vi "validate.vi"(8 "error in":errorcluster, 11 "Standard Engine Repo Data in":refnum<class "Standard Engine Configuration.lvclass">) -> (0 "error out":errorcluster, 3 "Standard Engine Repo Data out":refnum<class "Standard Engine Configuration.lvclass">)   [LabVIEW 2013, in "Standard Engine Configuration.lvclass"]
uses:
  Standard Engine Configuration.lvclass
  <vilib>/NI/Module Execution Interface/Engine Configuration/engine configuration.lvclass
  Standard Engine Configuration.lvclass/Standard Engine Configuration.ctl
  <vilib>/NI/CEF/CEF_TreeControl/NISE_CEF_TreeControl.lvlib
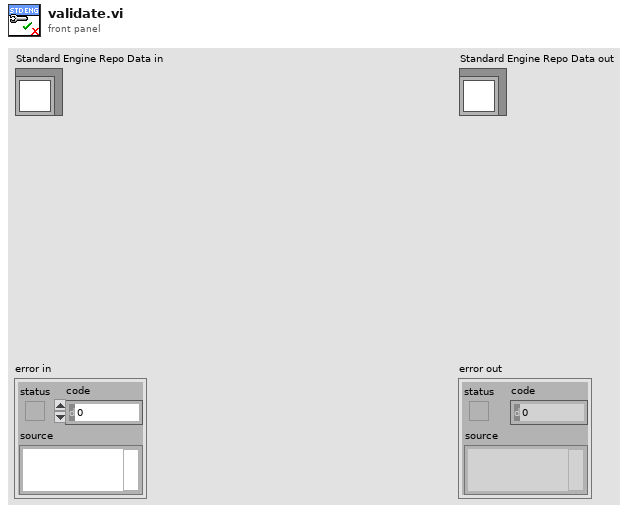
[diagram p1: front panel]
types:
  T1 = typedef "Standard Engine Configuration.lvclass/Module Specific Configuration.ctl" = cluster{"Module ID":string, "Module Decimation":T2, "Module Error Configuration":T3, "execution order priority":i32, "async?":bool, "error tag":string}
  T2 = typedef "Standard Engine Configuration.lvclass/Module Decimation.ctl" = cluster{"Decimation":u16, "Offset":u16}
  T3 = typedef "Standard Engine Configuration.lvclass/Module Error Configuration.ctl" = cluster{"Module Error Configuration":T4[]}
  T4 = typedef "Standard Engine Configuration.lvclass/Error Actions By Category.ctl" = cluster{"error classification":T5, "Error Actions":T6[]}
  T5 = typedef "TBM module execution interface.lvclass/error classification.ctl" = enum16{"unknown", "none", "trivial", "recoverable", "critical"}
  T6 = typedef "Standard Engine Configuration.lvclass/Error Actions.ctl" = enum16{"Clear", "Notify", "Stop Component", "Stop Engine", "Safe State", "Attempt Recovery"}
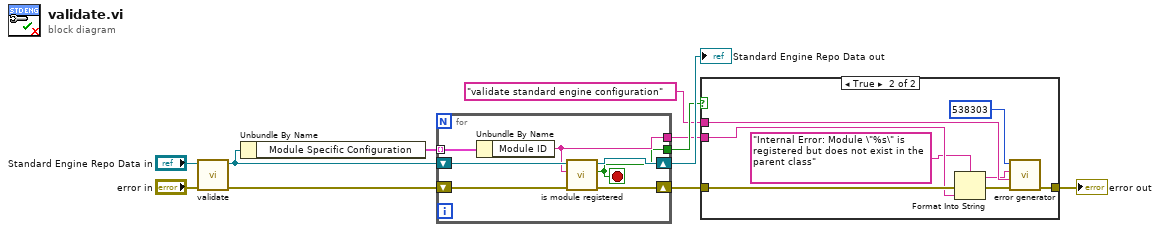
[diagram p0: block diagram]
diagram:
  n1 = call-parent "validate.vi"("error in"="error in", "configuration in"="Standard Engine Repo Data in") -> ("error out"=w7:errorcluster, "configuration out"=w9:refnum<class "Standard Engine Configuration.lvclass">)  [unwired: 8 in]
  n2 = Unbundle By Name(w9) -> ("Module Specific Configuration"=w6:T1[])
  n3 = for {
    shift-right: [w18] -> w8
    shift-left: w9 -> [w17]
    shift-right: [w15] -> w2
    shift-left: w7 -> [w16]
    tunnel: w6 -> [w14] mode=indexing
    tunnel: [w13] -> w3
    tunnel: [w12] -> w4
    stop <- w12 stop-if-true
    n4 = Unbundle By Name(w14) -> ("Module ID"=w13:string)
    n5 = call-dynamic "is module registered.vi"("error in"=w16, "module ID"=w13, "engine configuration in"=w17) -> ("error out"=w15:errorcluster, "registered?"=w12:bool, "engine configuration out"=w18:refnum<class "Standard Engine Configuration.lvclass">)  [unwired: 6 in]
  }
  "Standard Engine Repo Data out" <- w8
  n6 = case shown="True" w4 {
    tunnel: w2 -> [w19 w27]
    tunnel: [w19 w26] -> w5
    tunnel: "validate standard engine configuration" ("source") -> [_ w24]
    tunnel: w3 -> [_ w22]
    frame False {
    }
    frame True {
      n7 = Format Into String(format string="Internal Error: Module \"%s\" is registered but does not exist in the parent class", error in=w27, w22) -> (resulting string=w20:string, error out=w23:errorcluster)  [unwired: 1 in]
      n8 = call <vilib>:"error generator.vi"("error in"=w23, "source"=w24, "append error message"=w20, "error code (0)"=538303) -> ("error out"=w26:errorcluster)  [unwired: 5 in]
    }
  }
  "error out" <- w5
